vi "Find First Partial Matched Branch.vi"(8 "error in":errorcluster, 10 "Branch Name Pattern":string, 11 "Tree in":refnum<class "Tree.lvclass">) -> (0 "error out":errorcluster, 1 "Found?":bool, 2 "Matched Branch":refnum<class "Tree.lvclass">, 3 "Tree out":refnum<class "Tree.lvclass">)   [LabVIEW 2019, in "Tree.lvclass"]
uses:
  Tree.lvclass
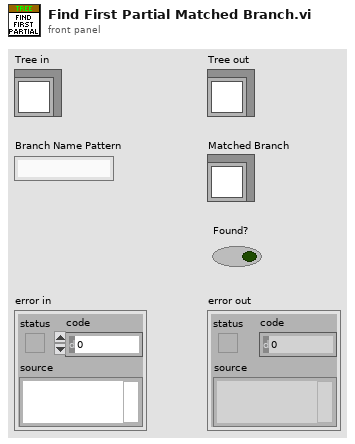
[diagram p1: front panel]
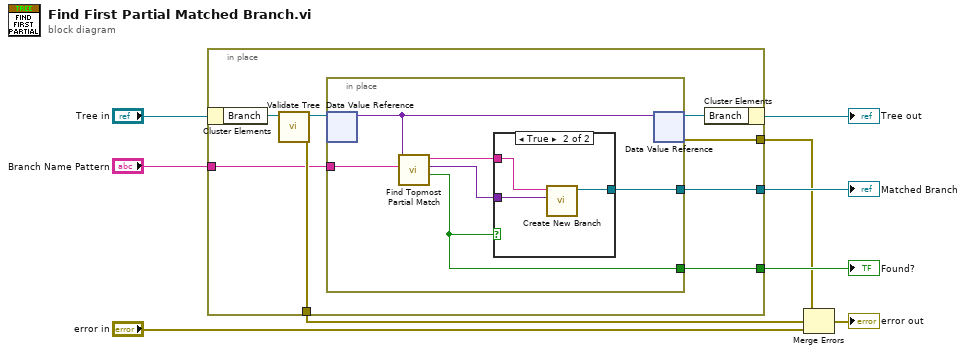
[diagram p0: block diagram]
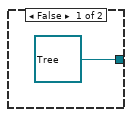
[diagram p2: hidden frame]
diagram:
  n1 = in-place {
    in-place-border: [w16] -> w1
    in-place-border: [w13] -> w5
    in-place-border: "Branch Name Pattern" -> [w12]
    in-place-border: [w11] -> w3
    in-place-border: [w10] -> w2
    n2 = in-place-cluster #1("Tree in") -> ("Branch"=w15:refnum<data-value>)
    n3 = call "Validate Tree.vi"("Branch Reference In"=w15) -> ("error out"=w13:errorcluster, "Branch Reference Out"=w14:refnum<data-value>)  [unwired: 9 in]
    n4 = in-place {
      in-place-border: w12 -> [w21]
      in-place-border: [w23] -> w11
      in-place-border: [w20] -> w10
      n5 = in-place-dvr #2(w14) -> (w22:variant)  [unwired: 1 out]
      n6 = call "Find Topmost Partial Match.vi"("Name"=w21, "Tree"=w22) -> ("Found?"=w20:bool, "Match"=w19:variant, "Node Name"=w18:string)  [unwired: 7 in]
      n7 = case shown="True" w20 {
        tunnel: w19 -> [_ w27]
        tunnel: [refnum<class "Tree.lvclass"> refnum ("Tree out") w26] -> w23
        tunnel: w18 -> [_ w25]
        frame False {
        }
        frame True {
          n8 = call "Create New Branch.vi"("Branch Data"=w27, "Name"=w25) -> ("Tree out"=w26:refnum<class "Tree.lvclass">)  [unwired: 8 in, 1 out]
        }
      }
      n9 = in-place-dvr #2(w22) -> (w17:refnum<data-value>, w16:errorcluster)
    }
    n10 = in-place-cluster #1("Branch"=w17) -> (→"Tree out":refnum<class "Tree.lvclass">)
  }
  "Matched Branch" <- w3
  "Found?" <- w2
  n11 = Merge Errors(w1, w5, "error in") -> (→"error out":errorcluster)
